vi "xyz from XYZ.vi"(0 "Data3D in":refnum<class "Data3D.lvclass">, 11 "error in (no error)":errorcluster) -> (4 "Data3D out":refnum<class "Data3D.lvclass">, 6 "x":dbl, 8 "y":dbl, 10 "z":dbl, 15 "error out":errorcluster)   [LabVIEW 2014, in "Data3D.lvclass"]
uses:
  Data3D.lvclass
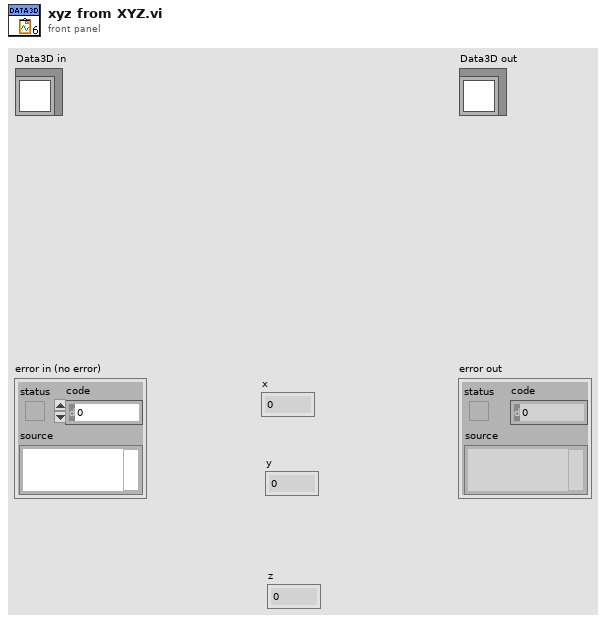
[diagram p1: front panel]
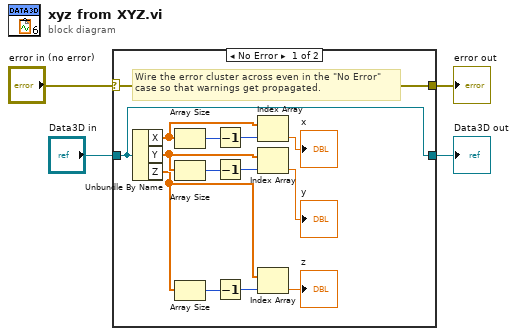
[diagram p0: block diagram]
diagram:
  n1 = case shown="No Error" "error in (no error)" {
    selector: "error in (no error)" -> [w18 w20]
    tunnel: [w18 w20] -> w3
    tunnel: [w8 w19] -> w1
    tunnel: "Data3D in" -> [w8 w19]
    frame No Error {
      # "Wire the error cluster across even in the \"No Error\"\ncase so that warnings get propagated."
      n2 = Unbundle By Name(w8) -> ("X"=w7:dbl[], "Y"=w6:dbl[], "Z"=w5:dbl[])
      n3 = Array Size(array=w7) -> (size(s)=w15:i32)
      n4 = Array Size(array=w6) -> (size(s)=w12:i32)
      n5 = Array Size(array=w5) -> (size(s)=w9:i32)
      n6 = Decrement(x=w15) -> (x-1=w16:i32)
      n7 = Decrement(x=w12) -> (x-1=w13:i32)
      n8 = Decrement(x=w9) -> (x-1=w10:i32)
      n9 = Index Array(array=w7, index=w16) -> (element=→"x":dbl)
      n10 = Index Array(array=w6, index=w13) -> (element=→"y":dbl)
      n11 = Index Array(array=w5, index=w10) -> (element=→"z":dbl)
    }
    frame Error {
    }
  }
  "error out" <- w3
  "Data3D out" <- w1
